vi "increment actor count.vi"(11 "Template in":refnum<class "Template.lvclass">) -> (3 "Template out":refnum<class "Template.lvclass">)   [LabVIEW 2020, in "Template.lvlib" / "Template.lvclass"]
doc: "Identifies the actor by a single, non-repeatable number.\nAll of the configurations from the Pre Launch Init.vi override should be done only by the actor 0!\nThe subsequential/channel-specific configurations should be done by the spawned actors.\nActor 0 does not return data!"
uses:
  Template.lvclass
  Template.lvclass/Template.ctl
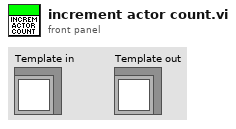
[diagram p1: front panel]
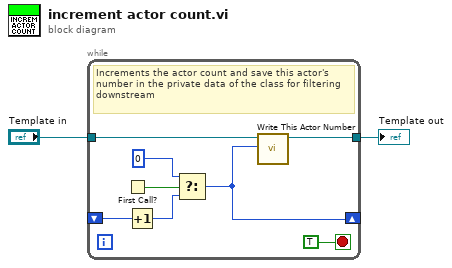
[diagram p0: block diagram]
diagram:
  n1 = while {
    tunnel: [w10] -> w2
    tunnel: "Template in" -> [w3]
    shift-right: [w8] -> _
    shift-left: _ -> [w7]
    stop <- TRUE stop-if-true
    # "Increments the actor count and save this actor's number in the private data of the class for filtering downstream"
    n2 = First Call?() -> (First Call?: T/F=w6:bool)
    n3 = Increment(x=w7) -> (x+1=w4:u32)
    n4 = Select(t=u32 0 ("This Actor Number"), s=w6, f=w4) -> (s? t:f=w8:u32)
    n5 = call "Write This Actor Number.vi"("This Actor Number"=w8, "Template in"=w3) -> ("Template out"=w10:refnum<class "Template.lvclass">)  [unwired: 9 in]
  }
  "Template out" <- w2
